vi "hWnd to U32.vi"(4 "hWnd":T1) -> (1 "hWnd":u32)   [LabVIEW 2011]
uses:
  hWnd.ctl
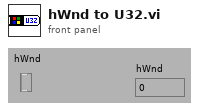
[diagram p1: front panel]
types:
  T1 = typedef "hWnd.ctl" = refnum<k1>
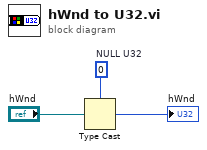
[diagram p0: block diagram]
diagram:
  w1 = u32 0  # NULL U32
  n1 = Type Cast(type=w1, x="hWnd") -> (*(type *) &x=→"hWnd":u32)
